vi "CRYGet Step Identify.vi"(8 "Unflatten Seq-step setup":string, 9 "Help?":bool, 10 "Value":string, 11 "Category Name In":string="stimulus.txt") -> (0 "Identfier":string="stimulus.txt", 1 "Identfier(*.)":string="stimulus.txt", 2 "Identfier(Regular Expression)":string="stimulus.txt", 3 "Category Name Out":string="stimulus.txt", 4 "Error?":bool, 5 "Symbol Index":i32, 6 "Help String":string, 7 "Project View Step Name Identifier":string)   [LabVIEW 2013]
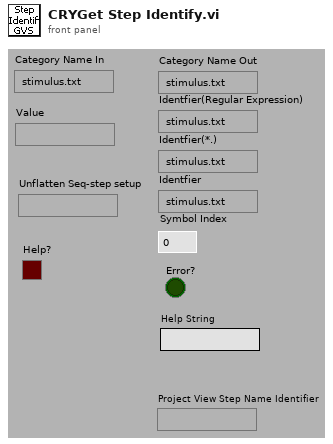
[diagram p1: front panel]
types:
  T1 = typedef "CRYAcquisition Cluster.ctl" = cluster{"Mode":u16, "Name":string, "use ch name":bool, "Record Time":dbl, "hide rec":bool, "hide play":bool, "rec delay":dbl, "rec pad":dbl, "dcc units":i8, "sine gen setting":string, "scope_fft setting":string, "voltmeter setting":string, "rta setting":string, "trig offset(sec)":dbl, "triggered  record":bool, "trig level":dbl, "trig unit":u8, "trig slop":bool, "trig timeout(sec)":dbl, "add record":bool, "EQ":bool, "record table":string[][], "play table":string[][], "trig channel":string, "Help":string}
  T2 = typedef "CRYAnalysis Cluster.ctl" = cluster{"Name":string, "Harmonics":dbl[], " Algorithm":u16, "delay":dbl, "THD(%)":bool, "Rub&Buzz":bool, "Imp":bool, "Imp Ref resistor":dbl, "Y data":u16, "Y prefix":string, "Y unit":string, "Y dB ref":dbl, "Custom Curve Names":string[], "har list items":string[], "Envelope":bool, "use custom unit":bool, "autodelay ch":dbl, "impulse":bool, " start ms":dbl, " stop ms":dbl, "Scaling":i32, "Default Overlap ":bool, "Advanced View":bool, "Loose Particle":bool, "Use default":bool, "Auto-Correlation(Stimulus)":bool, "Auto-Correlation(Response)":bool, "Deconvolved Response":bool, "Mic Current":bool, "M List Vaiues":u16, "Type":u16, "Delay Method":u16, "Apply Correction Out":bool, "Apply Correction In":bool, "Harmonics @ meas.frq":bool, "THD Normalized(%)":bool, "Total Distortion":bool, "THD+Noise(%)":bool, "Rub&Buzz Norm'd(%)":bool, "Standard Error":bool, "Confidence Limits":bool, "Total Diff":bool, "Total Noise":bool, "Total DFD(%)":bool, "Total IMD(%)":bool, "Total IM":bool, "Total DFD+Noise(%)":bool, "Use Channel Name":bool, "Waveform In":string, "Waveform Out":string, "Method":u16, "Spectral Scaling":u16, "Appliied Unit":u16, "Length Unit":u16, "Applied Units":u16, "Sens Item":u16, "Tab":i32, "Distance Unit":u16, "discard cycles":dbl, "Weigting":string, "Averaging Time":dbl, "Max duration":dbl, "Min duration":dbl, "Attack Threshold":dbl, "Hysteresis Up":dbl, "Fmin(Hz)":dbl, "Fmax(Hz)":dbl, "Freq.Resolution":dbl, "Over-samples Res.":dbl, "Win Resolution":dbl, "distance":dbl, "samples":dbl, "Overlap":dbl, "Record Length":dbl, "No.of FFTs":dbl, "Hz":dbl, "record delay":dbl, " Std Err":dbl, "Response":bool, "Coherent Power*":bool, "Stimulus":bool, "Measurement Confidence":bool, "Auto Spectrum(Response)*":bool, "Auto Spectrum(Stimulus)*":bool, "Cross Spectrum*":bool, "functions":bool, "Frequency Response":bool, "Non-Coherent Power*":bool, "Coherence (%)":bool, "Non-Coherence (%)":bool, "Signal-Noise Ratio (dB)":bool, "Non-Coherenct Distirtion*":bool, "Result Waveforms":bool, "Coupling":bool, "Averaging":u16, "Harmonics":i32, "Custom Curve Names":i32, "unLabel":string, "Custom Curve Names":string, "Unit":string, "Total IMD + Noise(%) ":bool, "ResponseMe":u16, "Intermod":dbl[], "Diff\n":dbl[], "Cross-Correlation":bool, "IM list items":string[], "Diff list items":string[], "TSR Window Type":string, "Help":string, "Custom Curve IDs":i32[], "Default Curve Names":string[], "Loose Particle waveform":bool, "Perceptual Rub&Buzz":bool, "Imp Auto Mode":u16, "Mic Auto Mode":u16, "Mic Ref resistor":dbl, "Curve Resolution":u16, "Curve Resolution Hz":dbl, "Polarity":bool}
  T3 = typedef "CRYAuto Save Cluster.ctl" = cluster{"Name":string, "save":enum16{"Data", "Results", "Waveforms"}, "Item Names":string[], "Autosave folder":path, "data format":u16, "filename option":enum16{"auto", "prompt"}, "fn construction":i32[], "layout":enum16{"rows", "columns"}, "notation":enum16{"sci", "float"}, "precision":i32, "prompt comment":bool, "header":enum16{"none", "standard", "custom"}, "custom header":string, "serial no.":bool, "User defined":string, "delimiter":enum16{"tab", "comma", "space", "other"}, "other delim":string, "axes":cluster{"x":bool, "y":bool, "z":bool}, "Time Stamp":bool, "Lot No.":bool, "Operator":bool, "Excel Template":string, "New or Append":u16, "Data":u16, "Help":string, "Tab Value":enum32{"Setting", "Help"}, "UDL or DSN":path, "User Default":bool, "Selector":i32, "Axis":u16, "Value Name":string, "format string":cluster{"dB Format String out":string, "Lin Format String out":string}, "DBPath":path}
  T4 = typedef "CRYCalibration All Cluster.ctl" = cluster{"Calibration 2D":T5[], "Help":string, "Tab Value":i32, "Input Signal Type":string, "Output Signal Type":string}
  T5 = typedef "CRYCalibration 2DCluster.ctl" = cluster{"Calibration":T6, "Corr Curve":T7, "EQ Curve":T7, "Sens Curve":T7}
  T6 = typedef "CRYCalibration Cluster.ctl" = cluster{"Calibration Step Name":string, "Device":string, "Correction Curve Name":string, "Equalization Curve Name":string, "Sensitivity Curve Name":string, "Corr Folder and File":string, "EQ Folder and File":string, "Sens Folder and File":string, "Corr Step size":u16, "EQ Step size":u16, "Input":bool, "Last Cal Date (sec)":timestamp, "Cha Name":string, "Corr Curve Found":bool, "EQ Curve Found":bool, "Sens Curve Found":bool, "Signal Type":string, "Calibrated Device":string, "Hz":u32}
  T7 = typedef "CRYData Cluster.ctl" = cluster{"Name":string, "Curve":cluster{"x":dbl, "y":dbl, "z":dbl}[], "X data":u16, "Y data":u16, "Z data":u16, "X axis":u16, "Y axis":u16, "Z axis":u16, "X unit":string, "Y unit":string, "Z unit":string, "X dB ref":dbl, "Y dB ref":dbl, "Z dB ref":dbl, "single val":bool, "protected":bool, "display X":bool, "display Y":bool, "display Z":bool, "Test Info":string, "Step No.":i32, "Plot Settings":cluster{"Color":u32, "Interpolation":u8, "Point Style":u8, "Line Style":u8, "Point Color":u32, "Line Width":u8, "Bar Plot Style":u8, "Fill To":i16}, "AutoProtect":bool}
  T8 = typedef "CRYHardware.ctl" = cluster{"Name":string, "Analog I/O":u16, "Digital I/O":u16, "Channels":u8, "Dig Dev ID":u8, "N ports":u8, "Interface":u32, "Dig I/O Ports":cluster{"port #":i16, "width":i16, "direction":i32}[], "Interf settings":cluster{"Type":u16, "COM Port":u8, "Baud rate":u32, "Data bits":u32, "Parity":u16, "Stop bits":u16, "Flow control":u16, "Dev ID IEEE":u8}[], "N interfs":i32, "udev SNs":i16[], "udev enable":bool, "Channel Array":T9[], "Cal sequence":string, "SelectedIn":u16, "SelectedOut":u16, "SelectedTab":u16, "State":bool, "Help":string, "Advanced":bool, "In Audio Driver":u16, "Out Audio Driver":u16}
  T9 = typedef "CRYHardware Channel Info.ctl" = cluster{"ID":i32, "Name":string, "Digital":bool, "Input":bool, "Device Name":string, "Hardware Ch ID":u8, "Vmax (V)":dbl, "Latency (samples)":dbl, "Sampling Rate (Hz)":u32, "Bit Depth":u32, "Anti-aliasing Factor (%fs)":sgl, "DAQmx Channel":tag, "term config":i32, "Coupling":i32, "IEPE en":bool, "ASIOChannel Name":string, "Audio Driver":u16, "ASIOChannel Index":u8}
  T10 = typedef "CRY6175Hardware.ctl" = cluster{"Tab Value":u16, "Help":string, "In Channel 1":u16, "In Channel 2":u16, "In Gain 1":i32, "In Gain 2":i32, "Mic Volt":i32, "Mic Resis":i32, "Out Channel":u16, "OUT_Impedance 1":u16, "OUT_Impedance 2":u16, "IN_Channel 1 Old":u16}
  T11 = typedef "CRYLimits.ctl" = cluster{"Name":string, "Tolerance":u16, "X Axis":u16, "Limits":u16, "Upper Limit":cluster{dbl, dbl}[], "Align Ref":cluster{dbl, dbl}, "Lower Limit":cluster{dbl, dbl}[], "Y data":u16, "Y unit":string, "Y dB ref":dbl, "Curve Names":string[], "Y-Resolution":u8, "Type":u16, "x float":bool, "X min-max-step":cluster{"Limit X Offset Min":dbl, "Limit X Offset Max":dbl, "Limit X Offset Step Size":dbl}, "magn/phase":u16, "Upper Limit Type":u16, "Lower Limit Type":u16, "Lim Curve axis up":u16, "Lim Curve axis lo":u16, "Data Selection Upper":u16, "Data Selection Lower":u16, "X-Resolution":u8, "Output failed point curves?":bool, "X data":u16, "X unit":string, "X dB ref":dbl, "X-Y Graph Set-up":string, "Tab Value":enum32{"Data", "Parameters"}, "Help":string, "X Up Val":dbl, "Y Up Val":dbl, "X Low Val":dbl, "Y Low Val":dbl, "Up Limit Val":dbl, "Low Limit Val":dbl, "bAdd DataName":bool, "Custom Name":string}
  T12 = typedef "CRYMessages Cluster.ctl" = cluster{"Name":string, "Type":u16, "Command Msg":string, "Flags":u16, "Dialog?":bool, "Numeric?":bool, "Wait?":bool, "Pause [ms]":i32, "pattern":u32, "Address":string, "Operation":i32, "bytes":i32, "Line selected":u32, "RS232 Func":u16, "Serial Ctrl lines":u16, "Interf #":u8, "GPIB func":u16, "GPIB cmd":u16, "GPIB rem en":bool, "GPIB term":i32, "Curves generated":string[], "Units":cluster{"unit":string, "dB ref":dbl, "axis":u16, "data":u16, "Common dB ref.":u16}, "Axis":u16, "Default Value":dbl, "Message Tilte":string, "Port #":i32, "Print Unit":string, "Text Format":cluster{"Size":u32, "Plain":bool, "Bold":bool, "Italic":bool, "Underline":bool, "Strikethrough":bool, "Color":u32, "Font":string}, "Help":string, "Tab Value":enum32{"Setting", "Help"}, "pattern 2":u32, "Line selected 2":u32, "H_Bits":cluster{"Bits":string[], "Invert":bool, "All":bool}[], "G_Bits":cluster{"Bits":string[], "Invert":bool, "All":bool}[]}
  T13 = typedef "CRYPost Processing Cluster.ctl" = cluster{"Name":string, "Op Type":u16, "Curve A":string, "Curve B":string, "Axis Mode":u16, "Work Mode":u16, "Width":u16, "Weighting win":u16, "Search Mode":u16, "Freq Mode":u16, "New Sampling Rate":dbl, "Use Default Name":bool, "x":bool, "y":bool, "z":bool, "All points":bool, "A_single val axis":u16, "B_single val axis":u16, "Use Default Value":bool, "Result Name":string, "Smoothing Width":i32, "Window":u16, "Para_dB":sgl, "Para_%":sgl, "Exponent":sgl, "Hz":dbl, "Direct Weighting":bool, "Auto Inc":bool, "Inc(deg)":i32, "Total Rotation":i32, "Ref Freq Mode":u16, "Ref Waveform":string, "Sampling Rate":dbl, "Weighting Curve":string, "Ref Freq":dbl, "Curve Group":string[], "Search Items":string[], "Custom unit info":cluster{"use custom":bool, "lin/log":u16, "unit":string, "dB ref":dbl, "common dB":u16}, "Unit":string, "Type A":enum16{"Curves", "Values", "Results", "WFM"}, "Type B":enum16{"Curves", "Values", "Results", "WFM"}, "Unary Operator":u16, "Binary Operator":u16, "Statistical Operator":u16, "Constant ":dbl, "New Resolution":u16, "user equation cluster":T14, "Help":string, "Tab Value":enum32{"Setting", "Help"}, "Zwciker_X-axis":u16, "Zwicker_spectrum":bool, "Freq Sampling Mode":u16, "Freq Sampling Rate":dbl, "Smoothing":bool, "Work in Statics":u16, "Result Data":string[]}
  T14 = typedef "CRYUser Equation Cluster.ctl" = cluster{"Custom unit input array":cluster{"use custom":bool, "lin/log":u16, "unit":string, "dB ref":dbl, "common dB":u16}[], "Custom unit results array ":cluster{"use custom":bool, "lin/log":u16, "unit":string, "dB ref":dbl, "common dB":u16}[], "Desired Result Variables":string[], "Desired Result Names":string[], "Input Curve Names":string[], "Input Curve Variables":string[], "equation":string, "Input axis":u16[], "Results axis":u16[], "# input curves":i32, "# Desired result curves ":i32, "Input Values":string[], "Result Values":string[]}
  T15 = typedef "CRYRecall Cluster.ctl" = cluster{"Name":string, "filepath":string, "all or last":i32, "File Path Mode":u16, "Curve Names":string[], "format string":cluster{"dB Format String out":string, "Lin Format String out":string}, "Template":u16[], "Axis":u16, "*.imp Path":path, "Filepath option":i16, "ML Value":dbl, "user defined":string, "Curves Selected?":bool[], "Help":string, "Tab Value":enum32{"Setting", "Help"}, "Selector":i32, "Use Default":bool}
  T16 = typedef "CRYStatistic cluster.ctl" = cluster{"Mode":u16, "No.Ranked(BF)":i32, "No.Ranked(WF)":i32, "Absolute Margin Standard Deviation":bool, "+/- sigma Res":i32, "Margin Standard Deviation":bool, "Margin Mean":bool, "Overall Yield":bool, "Individual Limits Yield":bool, "LSL Unit":string, "USL Unit\n":string, "LSL":dbl, "USL":dbl, "Worst Fit to Average":bool, "Best Fit to Average":bool, "Ppk":bool, "Pp":bool, "Absolute Standard Deviation":bool, "+/- sigma Dat":i32, "Standard Deviation ":bool, "Mean":bool, "Min ":bool, "Max ":bool, "No.of Curves Selected":i32, "Curves":string[], " Results":string[], "Name":string, "Help":string, "Tab Value":enum32{"Setting", "Help"}, "Work in":u16, "Mode xyz":u16}
  T17 = typedef "CRYSerial No.ctl" = cluster{"Name":string, "Mode":u16, "S/N prefix":string, "Tab Value":u16, "Help":string}
  T18 = typedef "CRYCustom Cluster.ctl" = cluster{"Help":string, "Flatten Data":string}
  T19 = typedef "CRYStimulus Cluster.ctl" = cluster{"StimulusType":string, "UseMLValArray":u16[], "ML_axisArray":u16[], "MLValLevelNameArray":string[], "Level(U)Array":dbl[], "Start(Stop)FreqArray":dbl[], "Start(Stop)AmpArray":dbl[], "StepResolutionArray":u16[], "Unit_Array":u16[], "DegValArray":dbl[], "DegUnitArray":string[], "Steps1":i32, "Cycle/step1(#)":u32, "Time/step1(s)":dbl, "Transition1":dbl, "SweepRate2":dbl, "Freq3(Hz)":dbl, "Steps3(#)":dbl, "Cycles3(#)":u32, "StepSize3":dbl, "wave time":string, "RMS_Value4":dbl, "Peak_Value4":dbl, "WavePath4":string, "RMS_unit4":string, "Peak_unit4":string, "wave Info":string, "dc_ctrl5_1":u16, "dc_ctrl5_2":u16, "dc_polar5":u16, "Max.Current":u16, "Steps5(#)":u32, "Time/Step5":dbl, "Level5":dbl, "StepsSize5Val":dbl, "StepSize5Unit":string, "SweepType":u16, "Fixed/Ratio6":u16, "Transition6":dbl, "Steps6(#)":dbl, "Cycle/Steps6(#)":u32, "Time/Steps6(s)":dbl, "Freq6(Hz)":dbl, "Difference6(Hz)":dbl, "Ratio6":string, "NoiseType7":u16, "Duration7(s)":dbl, "MinFreq7(Hz)":dbl, "MaxFreq7(Hz)":dbl, "MinFreq8(Hz)":dbl, "MaxFreq8(Hz)":dbl, "FreqRounding8":bool, "Duration8(s)":dbl, "Tones8":dbl, "RoundingVal8":dbl, "ApplyEQ":bool, "Duration(s)":dbl, "CustomStimulusName ":string, "Flatten Element Array":string[], "sine waves":cluster{"freq":dbl, "ampl":dbl, "cycles":dbl}[], "Channel Out":i32, "RatioVal6":dbl, "TabCtrl6":enum32{"Master Tone", "Slave Tone"}, "Signal Type Name":string, "Help":string, "Channel Sel":u16, "V on DUT":bool, "Output Imp":dbl, "Nominal Imp":dbl}
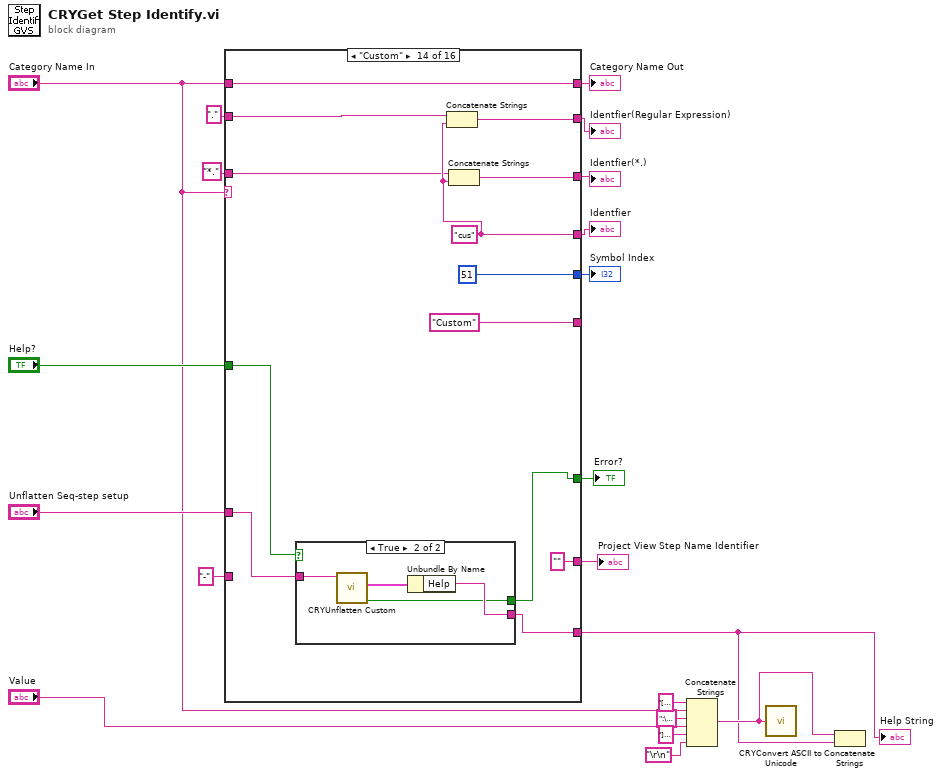
[diagram p0: block diagram]
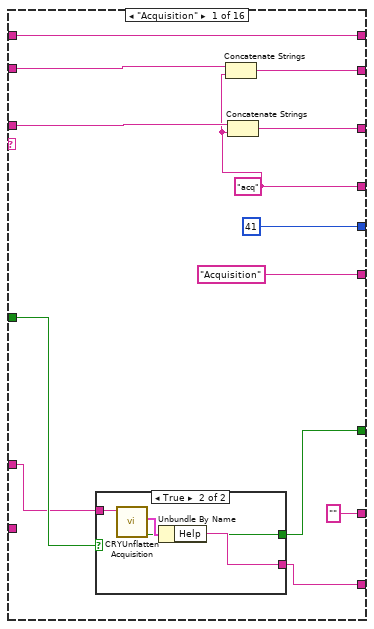
[diagram p2: hidden frame]
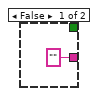
[diagram p3: hidden frame]
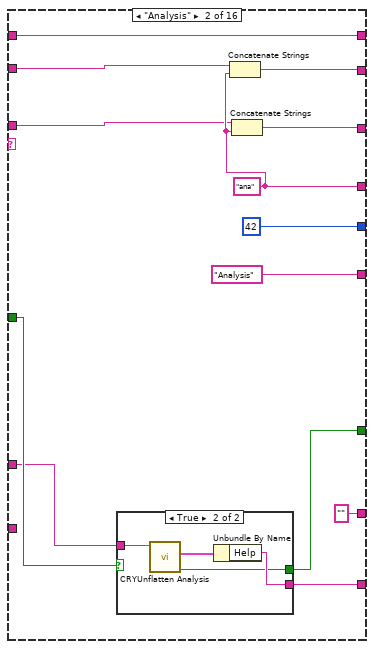
[diagram p4: hidden frame]
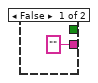
[diagram p5: hidden frame]
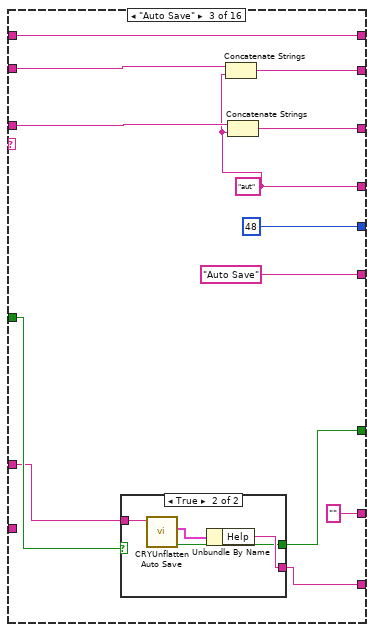
[diagram p6: hidden frame]
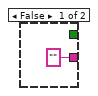
[diagram p7: hidden frame]
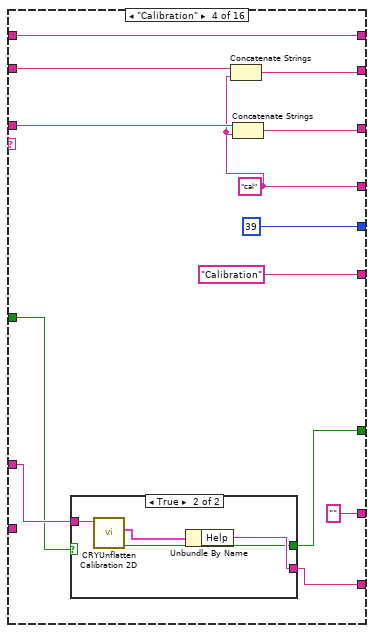
[diagram p8: hidden frame]
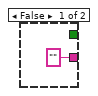
[diagram p9: hidden frame]
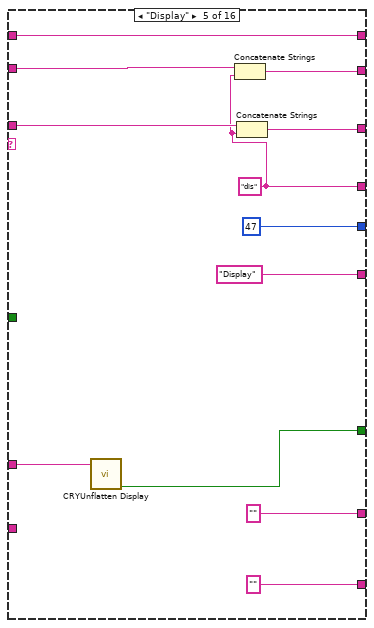
[diagram p10: hidden frame]
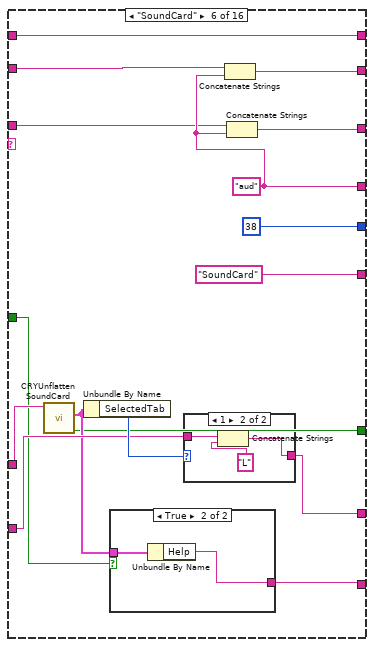
[diagram p11: hidden frame]
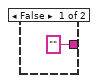
[diagram p12: hidden frame]
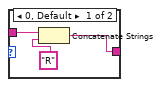
[diagram p13: hidden frame]
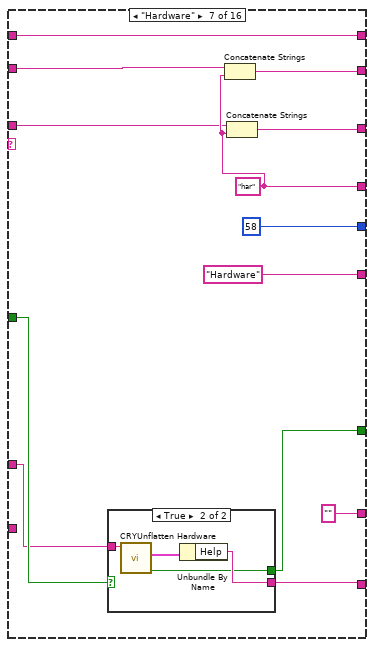
[diagram p14: hidden frame]
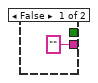
[diagram p15: hidden frame]
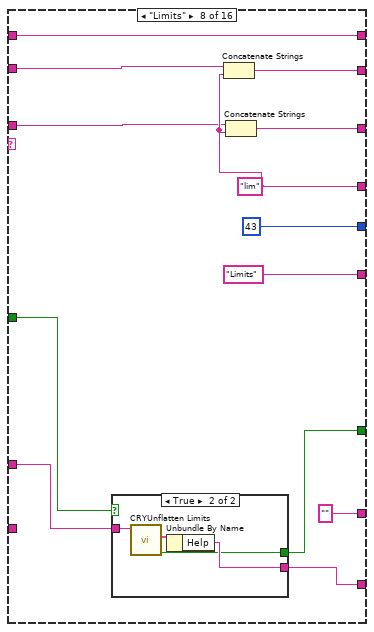
[diagram p16: hidden frame]
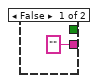
[diagram p17: hidden frame]
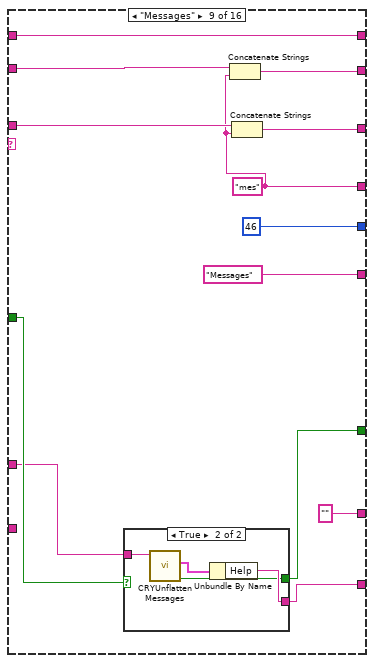
[diagram p18: hidden frame]
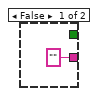
[diagram p19: hidden frame]
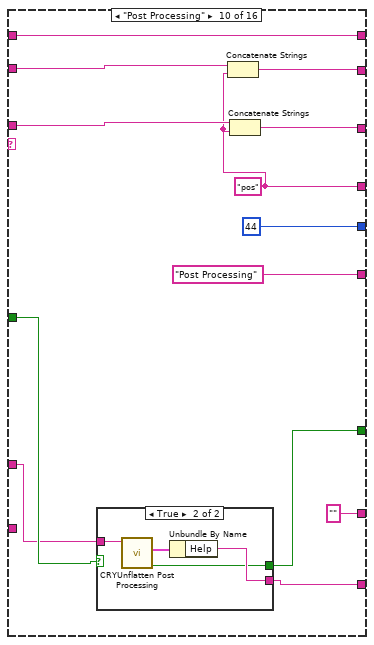
[diagram p20: hidden frame]
diagram:
  n1 = case shown="\"Custom\"" "Category Name In" {
    tunnel: [w26 w48 w62 w82 w97 w115 w137 w156 w171 w189 w207 w227 w245 w263 w282 "" ("Down Step Name")] -> w19
    tunnel: [w31 w49 w67 w85 w102 w118 w140 w158 w176 w194 w212 w230 w248 w266 w287 "" ("Down Step Name")] -> w20
    tunnel: ["Acquisition" ("Down Step Name") "Analysis" ("Down Step Name") "Auto Save" ("Down Step Name") "Calibration" ("Down Step Name") "Display" ("Down Step Name") "SoundCard" ("Down Step Name") "Hardware" ("Down Step Name") "Limits" ("Down Step Name") "Messages" ("Down Step Name") "Post Processing" ("Down Step Name") "Recall" ("Down Step Name") "Statistics" ("Down Step Name") "Serial No" ("Down Step Name") "Custom" ("Down Step Name") "Stimulus" ("Down Step Name") "" ("Down Step Name")] -> _
    tunnel: [41 ("Symbol Index") 42 ("Symbol Index") 48 ("Symbol Index") 39 ("Symbol Index") 47 ("Symbol Index") 38 ("Symbol Index") 58 ("Symbol Index") 43 ("Symbol Index") 46 ("Symbol Index") 44 ("Symbol Index") 49 ("Symbol Index") 45 ("Symbol Index") 50 ("Symbol Index") 51 ("Symbol Index") 40 ("Symbol Index") 37 ("Symbol Index")] -> w14
    tunnel: "Category Name In" -> [w31 w49 w67 w85 w102 w118 w140 w158 w176 w194 w212 w230 w248 w266 w287 _]
    tunnel: [w30 w45 w66 w80 w101 w117 w139 w157 w175 w193 w211 w229 w247 w265 w286 ""] -> w18
    tunnel: [w29 w44 w65 w81 w100 w116 w138 w153 w174 w192 w210 w228 w246 w264 w285 ""] -> w17
    tunnel: "." ("Down Step Name") -> [w27 w46 w63 w84 w98 w113 w135 w154 w172 w191 w208 w225 w243 w261 w284 _]
    tunnel: "*." ("Down Step Name") -> [w28 w47 w64 w83 w99 w114 w136 w155 w173 w190 w209 w226 w244 w262 w283 _]
    tunnel: "Unflatten Seq-step setup" -> [w22 w40 w58 w77 w94 w109 w132 w151 w168 w186 w203 w222 w240 w258 w281 _]
    tunnel: ["" "" "" "" "" w111 "" ("Help") "" "" "" "" "" "" "" w279 ""] -> w11
    tunnel: "-" ("Unflatten Seq-step setup") -> [_ _ _ _ _ w110 _ _ _ _ _ _ _ _ w280 _]
    tunnel: [w23 w42 w59 w78 "" ("Help String") w108 w134 w149 w167 w185 w205 w223 w241 w259 w275 "" ("Help String")] -> w1
    tunnel: "Help?" -> [w24 w41 w60 w76 _ w107 w133 w150 w169 w187 w204 w221 w239 w257 w277 _]
    tunnel: [w21 w39 w57 w75 w93 w105 w131 w148 w166 w184 w202 w220 w238 w256 w274 TRUE ("Error?")] -> w3
    frame "Acquisition" {
      w26 = "acq" ("Down Step Name")
      n2 = case shown="True" w24 {
        tunnel: ["" ("Help") w38] -> w23
        tunnel: w22 -> [_ w37]
        tunnel: [_ w35] -> w21
        frame False {
        }
        frame True {
          n3 = call "CRYUnflatten Acquisition.vi"("Flatten Acquisition"=w37) -> ("Error?"=w35:bool, "Acquisition"=w36:T1)  [unwired: 8 in, 1 out]
          n4 = Unbundle By Name(w36) -> ("Help"=w38:string)
        }
      }
      n5 = Concatenate Strings(w27, w26) -> (w30:string)
      n6 = Concatenate Strings(w28, w26) -> (w29:string)
    }
    frame "Analysis" {
      w48 = "ana" ("Down Step Name")
      n7 = case shown="True" w41 {
        tunnel: ["" ("Help") w56] -> w42
        tunnel: w40 -> [_ w55]
        tunnel: [_ w53] -> w39
        frame False {
        }
        frame True {
          n8 = call "CRYUnflatten Analysis.vi"("Unflatten Analysis"=w55) -> ("Error?"=w53:bool, "Analysis"=w54:T2)  [unwired: 8 in, 1 out]
          n9 = Unbundle By Name(w54) -> ("Help"=w56:string)
        }
      }
      n10 = Concatenate Strings(w46, w48) -> (w45:string)
      n11 = Concatenate Strings(w47, w48) -> (w44:string)
    }
    frame "Auto Save" {
      w62 = "aut" ("Down Step Name")
      n12 = case shown="True" w60 {
        tunnel: ["" ("Help") w74] -> w59
        tunnel: w58 -> [_ w73]
        tunnel: [_ w71] -> w57
        frame False {
        }
        frame True {
          n13 = call "CRYUnflatten Auto Save.vi"("Flatten Auto Save"=w73) -> ("Error?"=w71:bool, "Auto save"=w72:T3)  [unwired: 8 in, 1 out]
          n14 = Unbundle By Name(w72) -> ("Help"=w74:string)
        }
      }
      n15 = Concatenate Strings(w63, w62) -> (w66:string)
      n16 = Concatenate Strings(w64, w62) -> (w65:string)
    }
    frame "Calibration" {
      w82 = "cal" ("Down Step Name")
      n17 = case shown="True" w76 {
        tunnel: ["" ("Help") w92] -> w78
        tunnel: w77 -> [_ w91]
        tunnel: [_ w89] -> w75
        frame False {
        }
        frame True {
          n18 = call "CRYUnflatten Calibration 2D.vi"("Flattened Calibration"=w91) -> ("Error?"=w89:bool, "Calibration Step Out"=w90:T4)  [unwired: 8 in, 1 out]
          n19 = Unbundle By Name(w90) -> ("Help"=w92:string)
        }
      }
      n20 = Concatenate Strings(w84, w82) -> (w80:string)
      n21 = Concatenate Strings(w83, w82) -> (w81:string)
    }
    frame "Display" {
      w97 = "dis" ("Down Step Name")
      n22 = call "CRYUnflatten Display.vi"("Flatten Display"=w94) -> ("Error?"=w93:bool)  [unwired: 8 in, 2 out]
      n23 = Concatenate Strings(w98, w97) -> (w101:string)
      n24 = Concatenate Strings(w99, w97) -> (w100:string)
    }
    frame "SoundCard" {
      w115 = "aud" ("Down Step Name")
      n25 = call "CRYUnflatten SoundCard.vi"("Flatten SoundCard"=w109) -> ("Error?"=w105:bool, "SoundCard"=w106:T8)  [unwired: 9 out]
      n26 = Unbundle By Name(w106) -> ("SelectedTab"=w112:u16)
      n27 = case shown="True" w107 {
        tunnel: ["" ("Help") w122] -> w108
        tunnel: w106 -> [_ w123]
        frame False {
        }
        frame True {
          n28 = Unbundle By Name(w123) -> ("Help"=w122:string)
        }
      }
      n29 = case shown="1" w112 {
        tunnel: [w124 w127] -> w111
        tunnel: w110 -> [w126 w129]
        frame 0, Default {
          n30 = Concatenate Strings(w126, "R") -> (w124:string)
        }
        frame 1 {
          n31 = Concatenate Strings(w129, "L") -> (w127:string)
        }
      }
      n32 = Concatenate Strings(w113, w115) -> (w117:string)
      n33 = Concatenate Strings(w114, w115) -> (w116:string)
    }
    frame "Hardware" {
      w137 = "har" ("Down Step Name")
      n34 = case shown="True" w133 {
        tunnel: ["" ("Help") w147] -> w134
        tunnel: [_ w146] -> w131
        tunnel: w132 -> [_ w145]
        frame False {
        }
        frame True {
          n35 = call "CRYUnflatten Hardware.vi"("Unflatten Hardware#"=w145) -> ("Error?"=w146:bool, "Hardware"=w144:T10)  [unwired: 8 in, 1 out]
          n36 = Unbundle By Name(w144) -> ("Help"=w147:string)
        }
      }
      n37 = Concatenate Strings(w135, w137) -> (w139:string)
      n38 = Concatenate Strings(w136, w137) -> (w138:string)
    }
    frame "Limits" {
      w156 = "lim" ("Down Step Name")
      n39 = case shown="True" w150 {
        tunnel: ["" ("Help") w163] -> w149
        tunnel: w151 -> [_ w165]
        tunnel: [_ w162] -> w148
        frame False {
        }
        frame True {
          n40 = call "CRYUnflatten Limits.vi"("Unflatten Limits"=w165) -> ("Error?"=w162:bool, "Limits"=w164:T11)  [unwired: 8 in, 1 out]
          n41 = Unbundle By Name(w164) -> ("Help"=w163:string)
        }
      }
      n42 = Concatenate Strings(w154, w156) -> (w157:string)
      n43 = Concatenate Strings(w155, w156) -> (w153:string)
    }
    frame "Messages" {
      w171 = "mes" ("Down Step Name")
      n44 = case shown="True" w169 {
        tunnel: ["" ("Help") w183] -> w167
        tunnel: w168 -> [_ w182]
        tunnel: [_ w180] -> w166
        frame False {
        }
        frame True {
          n45 = call "CRYUnflatten Messages.vi"("Unflatten Messages"=w182) -> ("Error?"=w180:bool, "Messages"=w181:T12)  [unwired: 8 in, 1 out]
          n46 = Unbundle By Name(w181) -> ("Help"=w183:string)
        }
      }
      n47 = Concatenate Strings(w172, w171) -> (w175:string)
      n48 = Concatenate Strings(w173, w171) -> (w174:string)
    }
    frame "Post Processing" {
      w189 = "pos" ("Down Step Name")
      n49 = case shown="True" w187 {
        tunnel: ["" ("Help") w201] -> w185
        tunnel: w186 -> [_ w200]
        tunnel: [_ w198] -> w184
        frame False {
        }
        frame True {
          n50 = call "CRYUnflatten Post Processing.vi"("Unflatten Post Processing"=w200) -> ("Error?"=w198:bool, "Post-Processing"=w199:T13)  [unwired: 8 in, 1 out]
          n51 = Unbundle By Name(w199) -> ("Help"=w201:string)
        }
      }
      n52 = Concatenate Strings(w191, w189) -> (w193:string)
      n53 = Concatenate Strings(w190, w189) -> (w192:string)
    }
    frame "Recall" {
      w207 = "rec" ("Down Step Name")
      n54 = case shown="True" w204 {
        tunnel: ["" ("Help") w219] -> w205
        tunnel: w203 -> [_ w218]
        tunnel: [_ w216] -> w202
        frame False {
        }
        frame True {
          n55 = call "CRYUnflatten Recall.vi"("Flatten Recall"=w218) -> ("Error?"=w216:bool, "Recall setup"=w217:T15)  [unwired: 8 in, 1 out]
          n56 = Unbundle By Name(w217) -> ("Help"=w219:string)
        }
      }
      n57 = Concatenate Strings(w208, w207) -> (w211:string)
      n58 = Concatenate Strings(w209, w207) -> (w210:string)
    }
    frame "Statistics" {
      w227 = "sta" ("Down Step Name")
      n59 = case shown="True" w221 {
        tunnel: ["" ("Help") w236] -> w223
        tunnel: w222 -> [_ w237]
        tunnel: [_ w234] -> w220
        frame False {
        }
        frame True {
          n60 = call "CRYUnflatten Statistic.vi"("Flatten Statistics"=w237) -> ("Error?"=w234:bool, "Statistics"=w235:T16)  [unwired: 8 in, 1 out]
          n61 = Unbundle By Name(w235) -> ("Help"=w236:string)
        }
      }
      n62 = Concatenate Strings(w225, w227) -> (w229:string)
      n63 = Concatenate Strings(w226, w227) -> (w228:string)
    }
    frame "Serial No" {
      w245 = "ser" ("Down Step Name")
      n64 = case shown="False" w239 {
        tunnel: ["" ("Help") w254] -> w241
        tunnel: w240 -> [_ w255]
        tunnel: [_ w252] -> w238
        frame False {
        }
        frame True {
          n65 = call "CRYUnflatten Serial No.vi"("Unflatten Serial#"=w255) -> ("Error?"=w252:bool, "Serial#"=w253:T17)  [unwired: 8 in, 1 out]
          n66 = Unbundle By Name(w253) -> ("Help"=w254:string)
        }
      }
      n67 = Concatenate Strings(w243, w245) -> (w247:string)
      n68 = Concatenate Strings(w244, w245) -> (w246:string)
    }
    frame "Custom" {
      w263 = "cus" ("Down Step Name")
      n69 = case shown="True" w257 {
        tunnel: ["" ("Help") w272] -> w259
        tunnel: w258 -> [_ w273]
        tunnel: [_ w271] -> w256
        frame False {
        }
        frame True {
          n70 = call "CRYUnflatten Custom.vi"("Unflatten Custom"=w273) -> ("Error?"=w271:bool, "Custom"=w270:T18)  [unwired: 8 in, 1 out]
          n71 = Unbundle By Name(w270) -> ("Help"=w272:string)
        }
      }
      n72 = Concatenate Strings(w261, w263) -> (w265:string)
      n73 = Concatenate Strings(w262, w263) -> (w264:string)
    }
    frame "Stimulus" {
      w282 = "sti" ("Down Step Name")
      n74 = call "CRYUnflatten Stimulus.vi"("Flatten Stimulus"=w281) -> ("Error?"=w274:bool, "Stimulus"=w276:T19)  [unwired: 9 out]
      n75 = Unbundle By Name(w276) -> ("StimulusType"=w278:string)
      n76 = case shown="True" w277 {
        tunnel: w276 -> [_ w292]
        tunnel: ["" ("StimulusType") w291] -> w275
        frame False {
        }
        frame True {
          n77 = Unbundle By Name(w292) -> ("Help"=w291:string)
        }
      }
      n78 = Concatenate Strings(w280, w278) -> (w279:string)
      n79 = Concatenate Strings(w284, w282) -> (w286:string)
      n80 = Concatenate Strings(w283, w282) -> (w285:string)
    }
    frame Default {
    }
  }
  "Identfier" <- w19
  "Category Name Out" <- w20
  "Symbol Index" <- w14
  "Identfier(Regular Expression)" <- w18
  "Identfier(*.)" <- w17
  "Help String" <- w1
  "Project View Step Name Identifier" <- w11
  "Error?" <- w3
  n81 = Concatenate Strings("[\u0000" ("string"), "Category Name In", ":\u0000\u0000\u0000" ("string"), "Value", "]\u0000" ("string"), "\r\n") -> (w2:string)
  n82 = call "CRYConvert ASCII to Unicode.vi"("ASCII"=w2) -> ()  [unwired: 4 in, 1 out]
  n83 = Concatenate Strings(w2, w1) -> ()  [unwired: 1 out]
